vi "CTU.vi"(0 "CTU":bool, 2 "PV":i32, 3 "Reset":bool) -> (14 "Q":bool, 15 "CT":i32)   [LabVIEW 2020]
uses:
  7b58aaaf-3230-4726-a54c-2c8544926117.vi
panel:
  out "Mem":bool
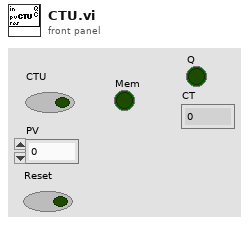
[diagram p1: front panel]
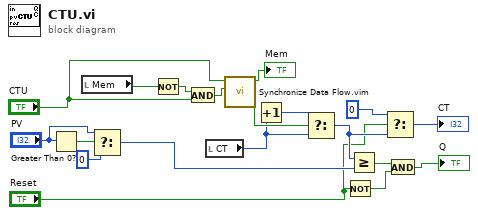
[diagram p0: block diagram]
diagram:
  n1 = Greater Than 0?(x="PV") -> (x > 0?=w19:bool)
  n2 = local read "Mem"() -> (w8:bool)
  n3 = Select(t="PV", s=w19, f=0) -> (s? t:f=w10:i32)
  n4 = Not(x=w8) -> (.not. x?=w9:bool)
  n5 = And(x=w9, y="CTU") -> (x .and. y?=w16:bool)
  n6 = local read "CT"() -> (w11:i32)
  n7 = call "Synchronize Data Flow.vim"("input 2"=w16, "input 1"="CTU") -> ("output 2"=w13:bool, "output 1"=→"Mem":bool)  [unwired: 2 in, 2 out]
  n8 = Increment(x=w11) -> (x+1=w12:i32)
  n9 = Select(t=w12, s=w13, f=w11) -> (s? t:f=w4:i32)
  n10 = Not(x="Reset") -> (.not. x?=w5:bool)
  n11 = Greater Or Equal?(x=w4, y=w10) -> (x >= y?=w7:bool)
  n12 = Select(t=0, s="Reset", f=w4) -> (s? t:f=→"CT":i32)
  n13 = And(x=w7, y=w5) -> (x .and. y?=→"Q":bool)
